vi "ReconnectDialog.vi"(8 "error in":errorcluster) -> (0 "error out":errorcluster, 3 "AbortConnection":bool)   [LabVIEW 2009]
panel:
  out "Message":string
  in  "Abort":bool
  in  "Reconnect":bool
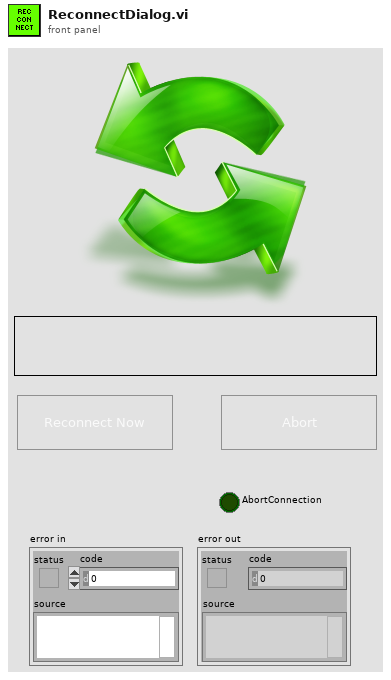
[diagram p1: front panel]
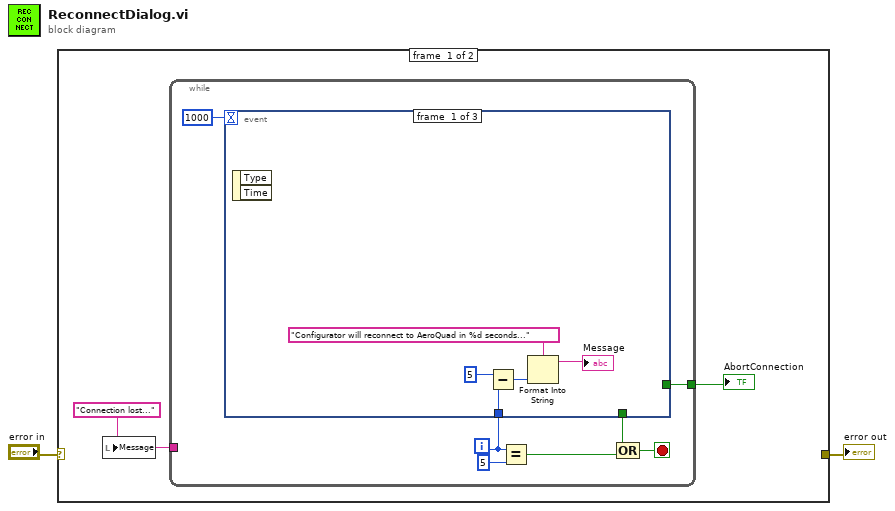
[diagram p0: block diagram]
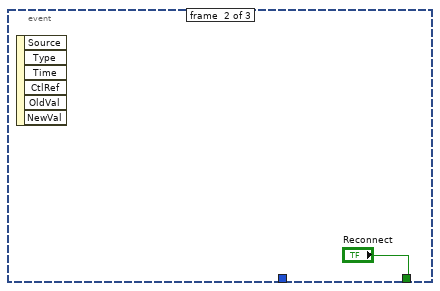
[diagram p2: hidden frame]
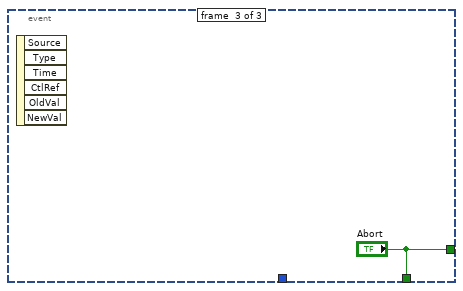
[diagram p3: hidden frame]
diagram:
  n1 = case shown="No Error" "error in" {
    selector: "error in" -> [_ w19]
    tunnel: [_ w19] -> w1
    frame #0 {
      w4 = "Connection lost..."
      n2 = local write "Message"(w4) -> ()
      n3 = while {
        tunnel: w4 -> [_]
        tunnel: [w5] -> w3
        i -> [w6]
        stop <- w8 stop-if-true
        n4 = event shown="[1] \"Reconnect\": Value Change" {
          selector: _ -> [_ _ _]
          dyn-events: _ -> [_ _ _]
          timeout: 1000 -> [_ _ _]
          tunnel: [_ "Reconnect" "Abort"] -> w7
          tunnel: w6 -> [w16 _ _]
          tunnel: [_ _ "Abort"] -> w5
          event #0 {
            n5 = event-data() -> ()  [unwired: 3 out]
            n6 = Subtract(x=5, y=w16) -> (x-y=w14:i32)
            n7 = Format Into String(format string="Configurator will reconnect to AeroQuad in %d seconds...", w14) -> (resulting string=→"Message":string)  [unwired: 2 in, 1 out]
          }
          event #1 {
            n8 = event-data() -> ()  [unwired: 7 out]
          }
          event #2 {
            n9 = event-data() -> ()  [unwired: 7 out]
          }
        }
        n10 = Equal?(x=w6, y=5) -> (x = y?=w9:bool)
        n11 = Compound Arithmetic op=OR(w7, w9) -> (w8:bool)
      }
      "AbortConnection" <- w3
    }
    frame #1 {
    }
  }
  "error out" <- w1
